vi "BRig_dataMTrig_Loop_T.vi"() -> (2 "output_Loop_T":i32)   [LabVIEW 2014]
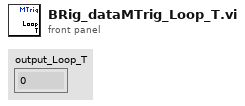
[diagram p1: front panel]
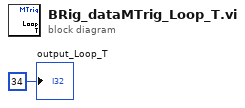
[diagram p0: block diagram]
diagram:
  "output_Loop_T" <- 34 ("output_iBlock")
